vi "Setup UI.vi"(8 "error in (no error)":errorcluster, 10 "Set UI to input? (F)":bool, 11 "Fluke Multimeter in":refnum<class "Fluke Multimeter.lvclass">) -> (0 "error out":errorcluster, 3 "Fluke Multimeter out":refnum<class "Fluke Multimeter.lvclass">)   [LabVIEW 2009, in "Fluke Multimeter.lvclass"]
doc: "Setup UI constructs an object -- populates its member fields -- from a front panel the user can see. The VI should be as simple as possible so that a UI loop can poll it continuously for updates. \n\nThe VI is designed to be used as a subPanel within another VI. Wire true to \"Set UI to input\" only on the first call, just after inserting this VI into a subPanel, to populate its controls with the class's current values.\n\nSetup UI is distinct from the class constructor. Class constructors are not polymorphic, yet configure dialogs need to configure objects without knowing their type -- and polymorphism is the necessary solution. Thus, Setup UI is a polymorphic class constructor. This continously polled \"Setup UI\" concept is a kludge: a better idea would be an XControl, but those require a steeper learning curve."
uses:
  Fluke Multimeter.lvclass
  Utility Classes/Readable/Readable.lvclass
  Fluke Multimeter.lvclass/Fluke Multimeter.ctl
panel:
  out "unit":string[](array[string])
  out "channel":string[](array[string])
  in  "trigger mode (0:internal)":u16(ring) items=["internal - continuous trigger", "external - rear panel trigger with delay", "external - bus trigger with delay", "external - rear panel trigger", "external - bus trigger"]
  in  "rate (0:slow)":u16(ring) items=["slow", "medium", "fast"]
  in  "range (0:auto)":u16(ring) items=["autorange", "200mV, 200 ohms", "2V, 2 kohms", "20V, 20 kohms", "200V, 200 kohms", "1000Vdc, 700 Vac, 2 Mohms", "20 Mohms"]
  in  "function (0:volts DC)":u16(ring) items=["volts DC", "volts AC", "2-wire k.ohms", "4-wire k.ohms", "mA DC", "mA AC"]
  # "Multimeter Setup"
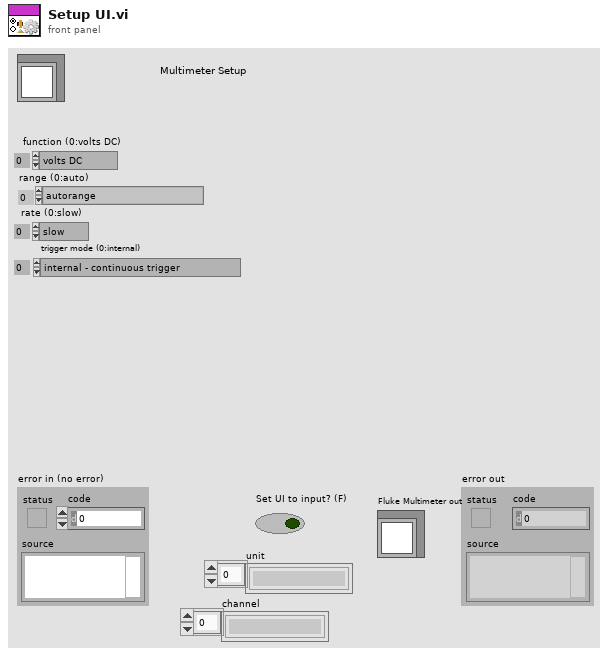
[diagram p1: front panel]
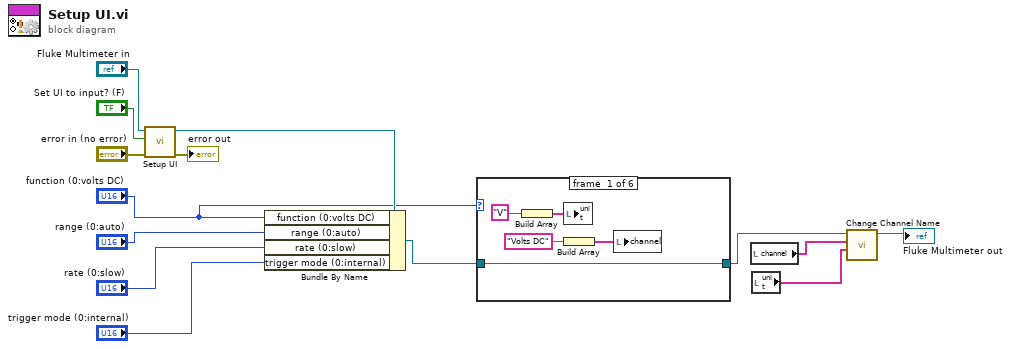
[diagram p0: block diagram]
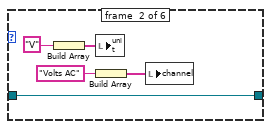
[diagram p2: hidden frame]
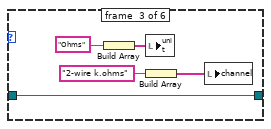
[diagram p3: hidden frame]
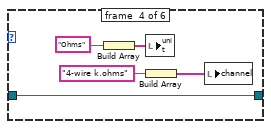
[diagram p4: hidden frame]
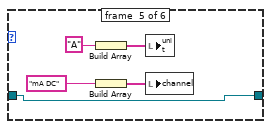
[diagram p5: hidden frame]
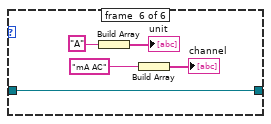
[diagram p6: hidden frame]
diagram:
  n1 = call-parent "Setup UI.vi"("error in (no error)"="error in (no error)", "Set UI to input? (F)"="Set UI to input? (F)", "Instrument in"="Fluke Multimeter in") -> ("error out"=→"error out":errorcluster, "Instrument out"=w10:refnum<class "Fluke Multimeter.lvclass">)  [unwired: 7 in]
  n2 = Bundle By Name(cluster=w10, "function (0:volts DC)"="function (0:volts DC)", "range (0:auto)"="range (0:auto)", "rate (0:slow)"="rate (0:slow)", "trigger mode (0:internal)"="trigger mode (0:internal)") -> (w5:refnum<class "Fluke Multimeter.lvclass">)
  n3 = case shown="0, Default" "function (0:volts DC)" {
    tunnel: w5 -> [w15 w20 w25 w30 w35 w40]
    tunnel: [w15 w20 w25 w30 w35 w40] -> w4
    frame #0 {
      n4 = Build Array("V") -> (w17:string[])
      n5 = local write "unit"(w17) -> ()
      n6 = Build Array("Volts DC") -> (w16:string[])
      n7 = local write "channel"(w16) -> ()
    }
    frame #1 {
      n8 = Build Array("V") -> (w21:string[])
      n9 = local write "unit"(w21) -> ()
      n10 = Build Array("Volts AC") -> (w22:string[])
      n11 = local write "channel"(w22) -> ()
    }
    frame #2 {
      n12 = Build Array("Ohms") -> (w26:string[])
      n13 = local write "unit"(w26) -> ()
      n14 = Build Array("2-wire k.ohms") -> (w27:string[])
      n15 = local write "channel"(w27) -> ()
    }
    frame #3 {
      n16 = Build Array("Ohms") -> (w31:string[])
      n17 = local write "unit"(w31) -> ()
      n18 = Build Array("4-wire k.ohms") -> (w32:string[])
      n19 = local write "channel"(w32) -> ()
    }
    frame #4 {
      n20 = Build Array("A") -> (w36:string[])
      n21 = Build Array("mA DC") -> (w37:string[])
      n22 = local write "unit"(w36) -> ()
      n23 = local write "channel"(w37) -> ()
    }
    frame #5 {
      n24 = Build Array("A") -> (→"unit":string[])
      n25 = Build Array("mA AC") -> (→"channel":string[])
    }
  }
  n26 = local read "channel"() -> (w2:string[])
  n27 = local read "unit"() -> (w1:string[])
  n28 = call "Change Channel Name.vi"("Channel Units"=w1, "Channel Names"=w2, "readable in"=w4) -> ("readable out"=→"Fluke Multimeter out":refnum<class "Fluke Multimeter.lvclass">)  [unwired: 8 in]
